vi "IsEqual.vi"(2 "is equal to":refnum<class "G#Object.lvclass">, 3 "reference in":refnum<class "G#Object.lvclass">) -> (0 "is equal":bool, 1 "reference out":refnum<class "G#Object.lvclass">)   [LabVIEW 2017, in "G#Object.lvclass"]
doc: "Checks if the two input object references are one and the same object."
uses:
  G#Object.lvclass
  G#Object.lvclass/G#Object.ctl
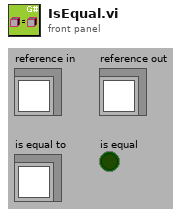
[diagram p1: front panel]
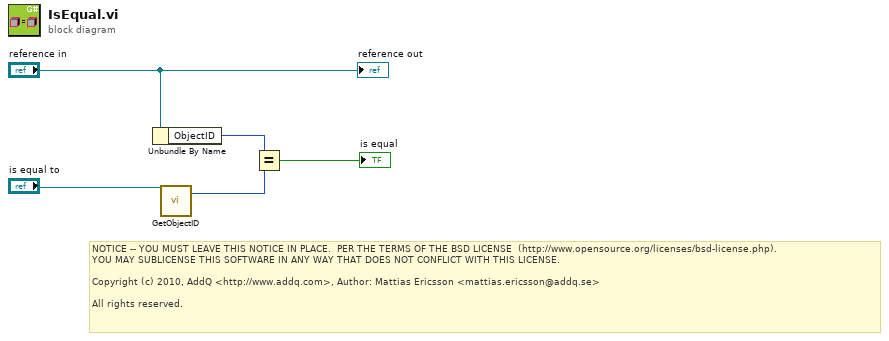
[diagram p0: block diagram]
diagram:
  # "NOTICE -- YOU MUST LEAVE THIS NOTICE IN PLACE.  PER THE TERMS OF THE BSD LICENSE  (http://www.opensource.org/licenses/bsd-license.php).\nYOU MAY SUBLICENSE THIS SOFTWARE IN ANY WAY THAT DOES NOT CONFLICT WITH THIS LICENSE.\n\nCopyright (c) 2010, AddQ <http://www.addq.com>, Author: Mattias Ericsson <mattias.ericsson@addq.se>\n\nAll rights reserved."
  n1 = Unbundle By Name("reference in") -> ("ObjectID"=w4:u32)
  n2 = call-dynamic "GetObjectID.vi"("reference in"="is equal to") -> ("object ID"=w1:u32)  [unwired: 16 in, 2 out]
  n3 = Equal?(x=w4, y=w1) -> (x = y?=→"is equal":bool)
  "reference out" <- "reference in"
